vi "LoadFrontPanelSettings.vi"(8 "error in (no error)":errorcluster, 11 "AutoModeData in":T1) -> (0 "error out":errorcluster, 3 "AutoModeData out":T1)   [LabVIEW 2019, in "AutoMode.lvlib"]
uses:
  AutoMode.lvlib
  Cluster - AutoModeData.ctl
  MainController/Cluster - TestSettings.ctl
  MainController/Cluster - HardwareConfiguration.ctl
  MainController/Cluster - TestResults.ctl
  Cluster - AutoModeMessage.ctl
  Enum - AutoModeState.ctl
  MainController/Cluster - MainControllerMessage.ctl
  MainController/Enum - MainState.ctl
  <vilib>/Utility/config.llb/Read Key (Boolean).vi
  <vilib>/Utility/config.llb/Read Key (Double).vi
  <vilib>/Utility/config.llb/Read Key (String).vi
  <vilib>/Utility/config.llb/Read Key (Path).vi
  <vilib>/Utility/config.llb/Read Key (I32).vi
  <vilib>/Utility/config.llb/NI_LVConfig.lvlib
  MainController/MainController.lvlib
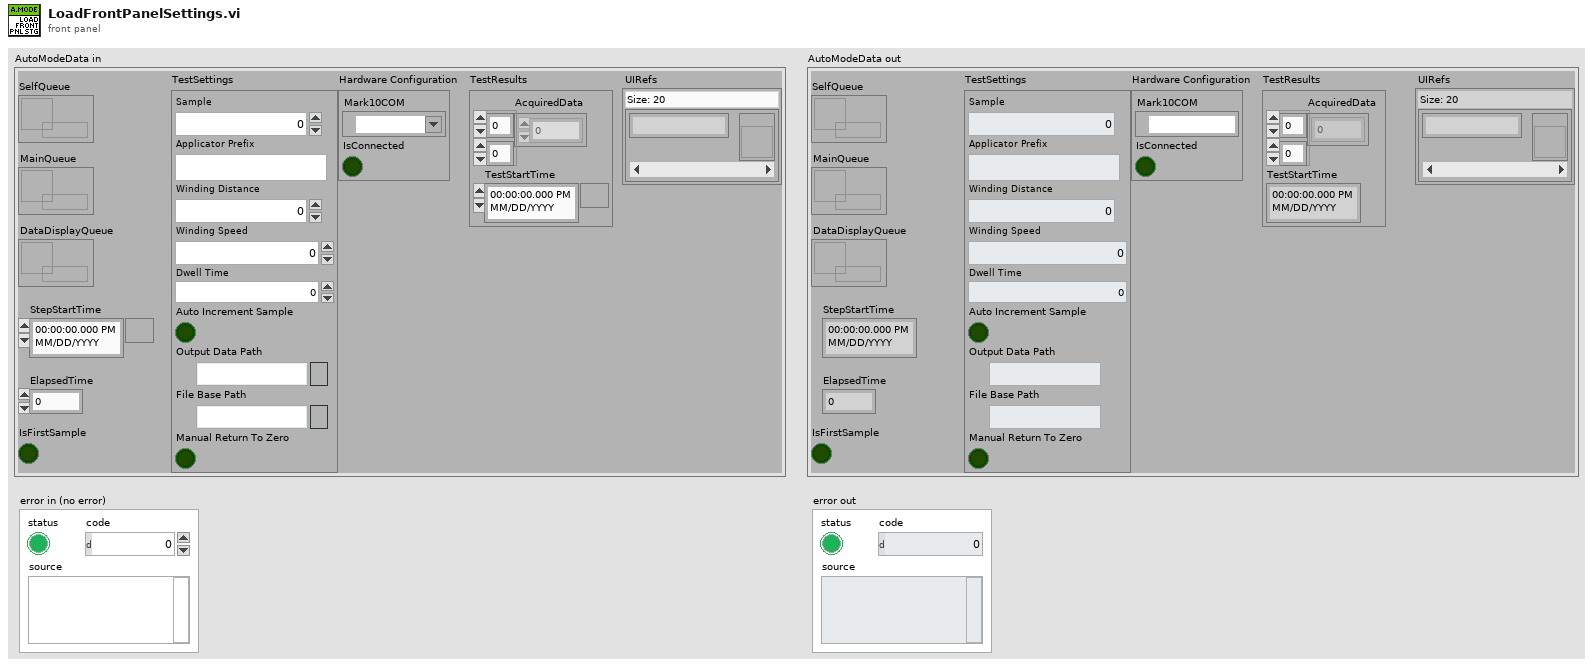
[diagram p1: front panel]
types:
  T1 = typedef "AutoMode.lvlib/Cluster - AutoModeData.ctl" = cluster{"DataDisplayQueue":refnum<queue>, "StepStartTime":timestamp, "TestSettings":T2, "Hardware Configuration":T3, "TestResults":T4, "ElapsedTime":dbl, "IsFirstSample":bool, "SelfQueue":refnum<queue>, "MainQueue":refnum<queue>, "UIRefs":map{string, refnum<vi>}}
  T2 = typedef "MainController.lvlib/Cluster - TestSettings.ctl" = cluster{"Sample":u32, "Applicator Prefix":string, "Winding Distance":dbl, "Winding Speed":dbl, "Dwell Time":dbl, "Auto Increment Sample":bool, "Output Data Path":path, "File Base Path":path, "Manual Return To Zero":bool}
  T3 = typedef "MainController.lvlib/Cluster - HardwareConfiguration.ctl" = cluster{"Mark10COM":refnum<visa-resource-name>, "IsConnected":bool}
  T4 = typedef "MainController.lvlib/Cluster - TestResults.ctl" = cluster{"AcquiredData":dbl[][], "TestStartTime":timestamp}
  T5 = enum32{"0 <undefined>", "1 <undefined>", "2 <undefined>", "Generic", "Decoration", "Text", "Control", "ColorBox", "Boolean", "RefNum", "Variant", "Path", "ListBox", "Table", "Array", "Picture", "ActiveXContainer", "Numeric", "Digital", "NamedNumeric", "ColorRamp", "Slide", "GraphOrChart", "WaveformChart", "WaveformGraph", "IntensityChart", "IntensityGraph", "String", "IOName", "ComboBox", "Cluster", "Panel", "Knob", "NumWithScale", "Ring", "Enum", "GObject", "Plot", "Cursor", "NumericText", "Scale", "ColorScale", "GraphScale", "ColorGraphScale", "TypedRefNum", "OldKnobScale", "MCListbox", "MeasureData", "BVTag", "DAQName", "VISAName", "IVIName", "SlideScale", "TabControl", "Page", "TabArrayTabControl", "ConPane"}
  T6 = typedef "NI_LVConfig.lvlib/Config Data RefNum.ctl" = refnum<k1>
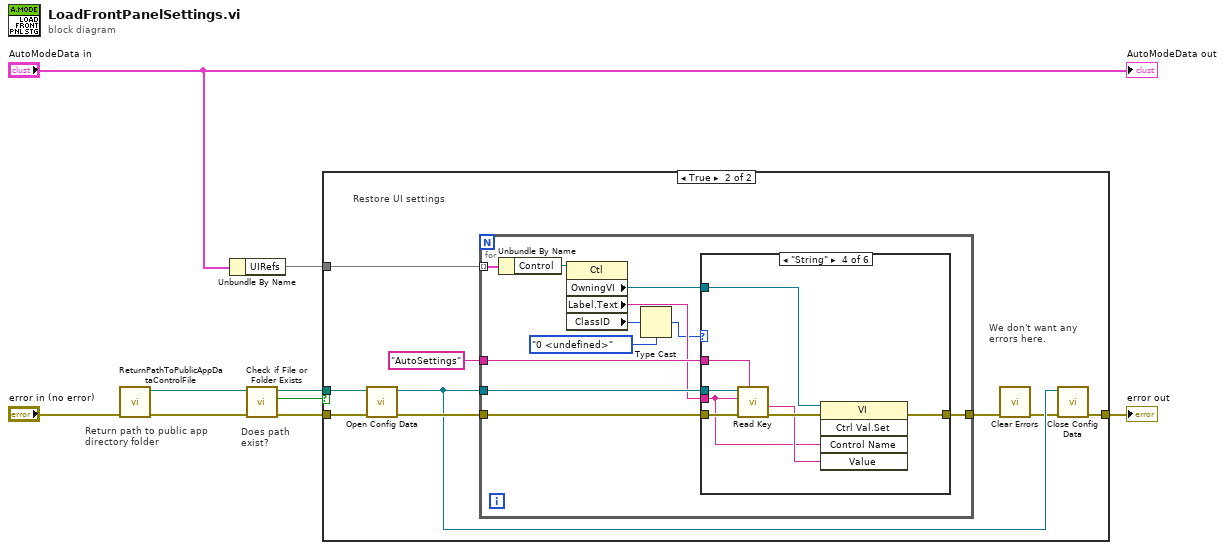
[diagram p0: block diagram]
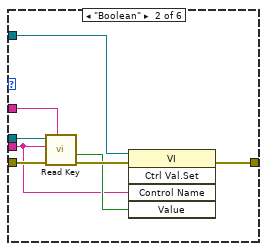
[diagram p4: hidden frame]
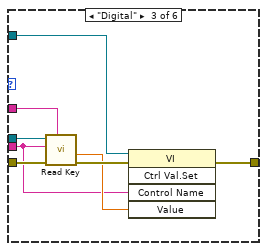
[diagram p5: hidden frame]
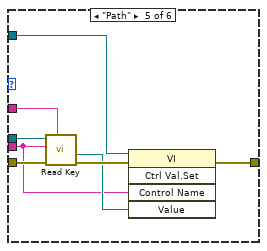
[diagram p6: hidden frame]
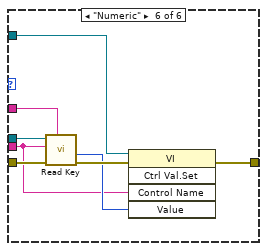
[diagram p7: hidden frame]
diagram:
  # "Return path to public app directory folder"
  # "Does path\nexist?"
  n1 = call "ReturnPathToPublicAppDataControlFile.vi"("error in (no error)"="error in (no error)") -> ("error out"=w8:errorcluster, "UIControlsFilePath"=w4:path)  [unwired: 9 in]
  n2 = Unbundle By Name("AutoModeData in") -> ("UIRefs"=w1:map{string, refnum<vi>})
  n3 = call <vilib>:"Check if File or Folder Exists.vi"("error in (no error)"=w8, "path"=w4) -> ("error out"=w5:errorcluster, "file or folder exists?"=w2:bool, "dup path"=w3:path)  [unwired: 7 in]
  n4 = case shown="True" w2 {
    tunnel: [w10 w13] -> w6
    tunnel: w5 -> [w10 w19]
    tunnel: w3 -> [_ w18]
    tunnel: w1 -> [_ w17]
    frame False {
    }
    frame True {
      # "We don't want any\nerrors here."
      # "Restore UI settings"
      n5 = call <vilib>:"Open Config Data.vi"("error in (no error)"=w19, "configuration file path"=w18) -> ("error out"=w16:errorcluster, "refnum"=w12:T6)  [unwired: 7 in, 1 out]
      n6 = for {
        tunnel: w17 -> [w30] mode=indexing
        tunnel: w12 -> [w27]
        tunnel: "AutoSettings" ("section") -> [w26]
        tunnel: w16 -> [w28]
        tunnel: [w20] -> w15
        n7 = Unbundle By Name(w30) -> ("Control"=w29:refnum<vi>)
        n8 = property class="Ctl"(reference=w29) -> ("OwningVI"=w21:refnum<vi>, "Label.Text"=w23:string, "ClassID"=w25:u32)  [unwired: 1 in, 2 out]
        n9 = Type Cast(type=T5."0 <undefined>" ("ClassID Name"), x=w25) -> (*(type *) &x=w22:T5)
        n10 = case shown="\"String\"" w22 {
          tunnel: w28 -> [w31 w39 w47 w55 w63 w71]
          tunnel: w27 -> [_ w38 w46 w54 w62 w70]
          tunnel: w26 -> [_ w37 w45 w53 w61 w69]
          tunnel: w23 -> [_ w34 w42 w50 w58 w66]
          tunnel: w21 -> [_ w33 w41 w49 w57 w65]
          tunnel: [w31 w32 w40 w48 w56 w64] -> w20
          frame "0 <undefined>", Default {
          }
          frame "Boolean" {
            n11 = call-poly <vilib>:"Read Key.vi"("section"=w37, "error in (no error)"=w39, "key"=w34, "refnum"=w38) -> ("error out"=w36:errorcluster, "value"=w35:bool)  [unwired: 4 in, 2 out]
            n12 = invoke class="VI" method="Ctrl Val.Set"(reference=w33, error in=w36, "Control Name"=w34, "Value"=w35) -> (error out=w32:errorcluster)  [unwired: 1 in, 4 out]
          }
          frame "Digital" {
            n13 = call-poly <vilib>:"Read Key.vi"("section"=w45, "error in (no error)"=w47, "key"=w42, "refnum"=w46) -> ("error out"=w44:errorcluster, "value"=w43:dbl)  [unwired: 4 in, 2 out]
            n14 = invoke class="VI" method="Ctrl Val.Set"(reference=w41, error in=w44, "Control Name"=w42, "Value"=w43) -> (error out=w40:errorcluster)  [unwired: 1 in, 4 out]
          }
          frame "String" {
            n15 = call-poly <vilib>:"Read Key.vi"("section"=w53, "error in (no error)"=w55, "key"=w50, "refnum"=w54) -> ("error out"=w52:errorcluster, "value"=w51:string)  [unwired: 4 in, 2 out]
            n16 = invoke class="VI" method="Ctrl Val.Set"(reference=w49, error in=w52, "Control Name"=w50, "Value"=w51) -> (error out=w48:errorcluster)  [unwired: 1 in, 4 out]
          }
          frame "Path" {
            n17 = call-poly <vilib>:"Read Key.vi"("section"=w61, "error in (no error)"=w63, "key"=w58, "refnum"=w62) -> ("error out"=w60:errorcluster, "value"=w59:path)  [unwired: 4 in, 2 out]
            n18 = invoke class="VI" method="Ctrl Val.Set"(reference=w57, error in=w60, "Control Name"=w58, "Value"=w59) -> (error out=w56:errorcluster)  [unwired: 1 in, 4 out]
          }
          frame "Numeric" {
            n19 = call-poly <vilib>:"Read Key.vi"("section"=w69, "error in (no error)"=w71, "key"=w66, "refnum"=w70) -> ("error out"=w68:errorcluster, "value"=w67:i32)  [unwired: 4 in, 2 out]
            n20 = invoke class="VI" method="Ctrl Val.Set"(reference=w65, error in=w68, "Control Name"=w66, "Value"=w67) -> (error out=w64:errorcluster)  [unwired: 1 in, 4 out]
          }
        }
      }
      n21 = call <vilib>:"Clear Errors.vi"("error in (no error)"=w15) -> ("error out"=w11:errorcluster)  [unwired: 5 in, 1 out]
      n22 = call <vilib>:"Close Config Data.vi"("error in (no error)"=w11, "refnum"=w12) -> ("error out"=w13:errorcluster)  [unwired: 8 in, 1 out]
    }
  }
  "error out" <- w6
  "AutoModeData out" <- "AutoModeData in"
